vi "Assign HS Master Timing.vi"(8 "error in (no error)":errorcluster, 11 "DAQ Task in":refnum<class "DAQ Task.lvclass">) -> (0 "error out":errorcluster, 2 "MasterTimingInfo":T1, 3 "DAQ Task out":refnum<class "DAQ Task.lvclass">)   [LabVIEW 2012, in "Data Acquisition.lvlib" / "DAQ Task.lvclass"]
uses:
  DAQ Task.lvclass
  Controls/Master Timing Info.ctl
  DAQ Task.lvclass/DAQ Task.ctl
  <resource>/objmgr/daqmx.rc
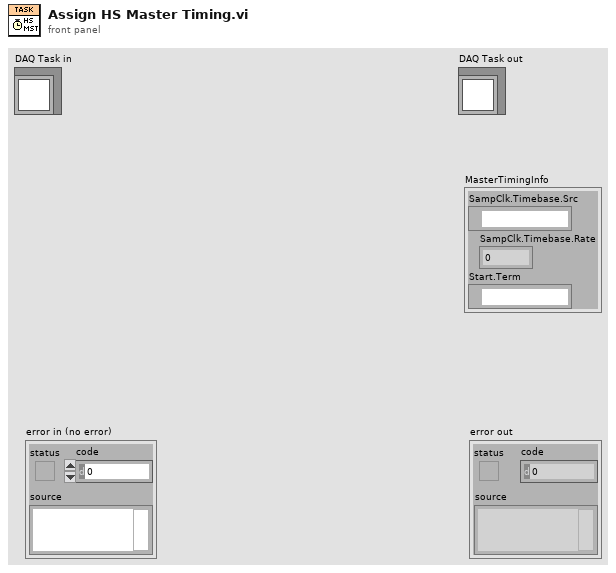
[diagram p1: front panel]
types:
  T1 = typedef "Data Acquisition.lvlib/DAQ Task.lvclass/Master Timing Info.ctl" = cluster{"SampClk.Timebase.Src":tag, "SampClk.Timebase.Rate":dbl, "Start.Term":tag}
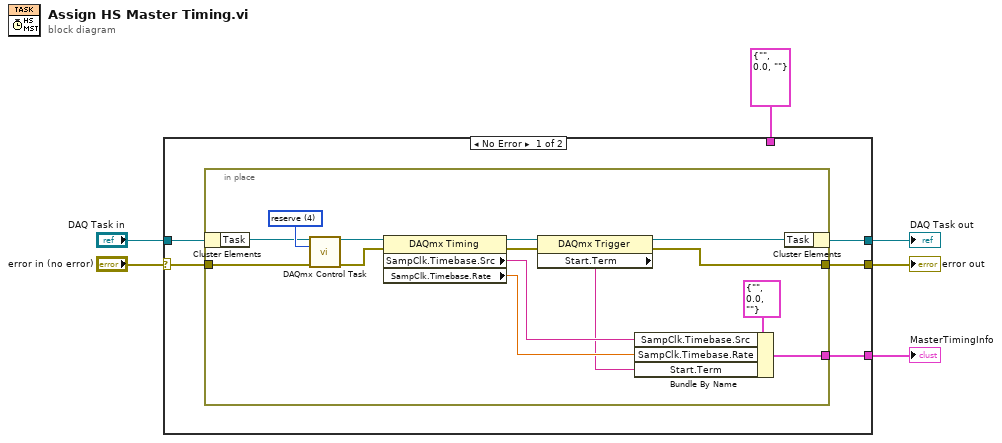
[diagram p0: block diagram]
diagram:
  n1 = case shown="No Error" "error in (no error)" {
    selector: "error in (no error)" -> [w7 w28]
    tunnel: [w11 w28] -> w5
    tunnel: [w9 w27] -> w3
    tunnel: "DAQ Task in" -> [w8 w27]
    tunnel: [w10 w26] -> w2
    tunnel: T1 {"SampClk.Timebase.Src"="", "SampClk.Timebase.Rate"=0.0, "Start.Term"=""} ("MasterTimingInfo") -> [_ w26]
    frame No Error {
      n2 = in-place {
        in-place-border: [w25] -> w11
        in-place-border: [w24] -> w10
        in-place-border: w7 -> [w14]
        w23 = 4 items=["verify"=2, "reserve"=4, "commit"=3, "unreserve"=5, "abort"=6] ("action")
        n3 = in-place-cluster #1(w8) -> ("Task"=w12:refnum<k21>)
        n4 = call <vilib>:"DAQmx Control Task.vi"("task/channels in"=w12, "action"=w23, "error in"=w14) -> ("task out"=w22:refnum<k21>, "error out"=w19:errorcluster)  [unwired: 11 in]
        n5 = property class="DAQmx Timing"(reference=w22, error in=w19) -> (reference out=w21:refnum<k21>, error out=w20:errorcluster, "SampClk.Timebase.Src"=w17:tag, "SampClk.Timebase.Rate"=w16:dbl)
        n6 = property class="DAQmx Trigger"(reference=w21, error in=w20) -> (reference out=w13:refnum<k21>, error out=w25:errorcluster, "Start.Term"=w15:tag)
        n7 = Bundle By Name(cluster=T1 {"SampClk.Timebase.Src"="", "SampClk.Timebase.Rate"=0.0, "Start.Term"=""} ("MasterTimingInfo"), "SampClk.Timebase.Src"=w17, "SampClk.Timebase.Rate"=w16, "Start.Term"=w15) -> (w24:T1)
        n8 = in-place-cluster #1("Task"=w13) -> (w9:refnum<class "DAQ Task.lvclass">)
      }
    }
    frame Error {
    }
  }
  "error out" <- w5
  "DAQ Task out" <- w3
  "MasterTimingInfo" <- w2
